vi "Fs(Hz), T(ms) to Fs, Samples.vi"(5 "Duration (ms)":dbl, 6 "Sampling rate (Hz)":dbl) -> (1 "Samples":i32, 2 "Sampling rate (Hz) Out":dbl)   [LabVIEW 2020]
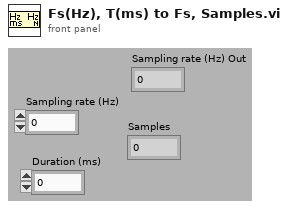
[diagram p1: front panel]
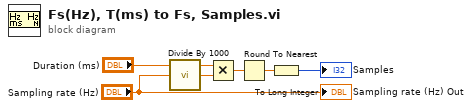
[diagram p0: block diagram]
diagram:
  n1 = call "Divide By 1000.vi"("X"="Sampling rate (Hz)") -> ("X/1000"=w1:dbl)
  n2 = Multiply(x="Duration (ms)", y=w1) -> (x*y=w4:dbl)
  n3 = Round To Nearest(number=w4) -> (nearest integer value=w3:dbl)
  n4 = To Long Integer(number=w3) -> (32bit integer=→"Samples":i32)
  "Sampling rate (Hz) Out" <- "Sampling rate (Hz)"
